vi "Sending U8x2 CMD and String Data.vi"(0 "TCP Ref In":refnum<k5>, 1 "Time Out(ms)":i32=100, 5 "High CMD":u8, 7 "Low CMD":u8, 9 "Data":string, 11 "error in (no error)":errorcluster) -> (4 "TCP Ref Out":refnum<k5>, 15 "error out":errorcluster)   [LabVIEW 2024]
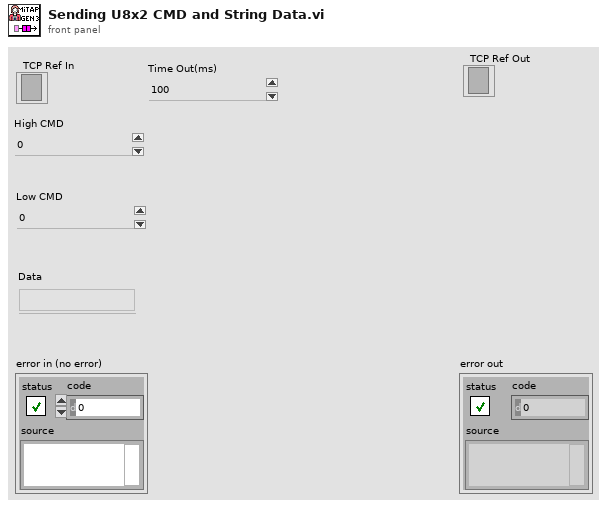
[diagram p1: front panel]
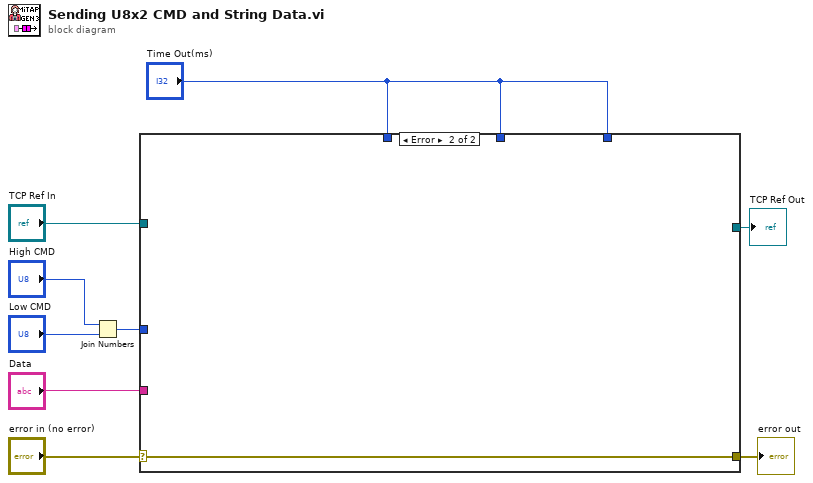
[diagram p0: block diagram]
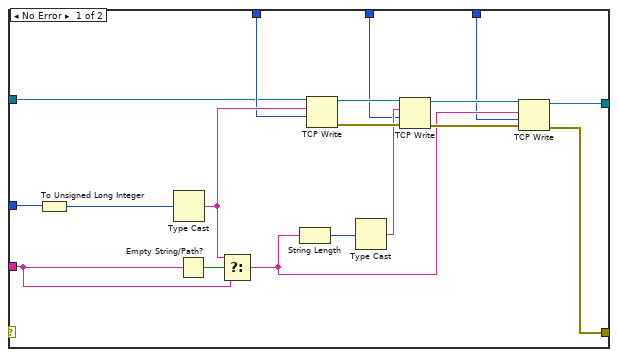
[diagram p2: hidden frame]
diagram:
  n1 = Join Numbers(hi="High CMD", lo="Low CMD") -> ((hi.lo)=w5:u16)
  n2 = case shown="Error" "error in (no error)" {
    selector: "error in (no error)" -> [_ w28]
    tunnel: [w18 w28] -> w9
    tunnel: "Time Out(ms)" -> [w17 _]
    tunnel: "Time Out(ms)" -> [w16 _]
    tunnel: "Time Out(ms)" -> [w15 _]
    tunnel: "TCP Ref In" -> [w14 _]
    tunnel: [w13 _] -> w6
    tunnel: w5 -> [w12 _]
    tunnel: "Data" -> [w10 _]
    frame No Error {
      n3 = To Unsigned Long Integer(number=w12) -> (unsigned 32bit integer=w11:u32)
      n4 = Type Cast(x=w11) -> (*(type *) &x=w20:string)  [unwired: 1 in]
      n5 = Empty String/Path?(string/path=w10) -> (empty?=w21:bool)
      n6 = Select(t=w20, s=w21, f=w10) -> (s? t:f=w19:string)
      n7 = String Length(string=w19) -> (length=w23:i32)
      n8 = TCP Write(connection ID=w14, data in=w20, 9:w17) -> (connection ID out=w27:refnum<k5>, error out=w26:errorcluster)  [unwired: 1 in, 1 out]
      n9 = Type Cast(x=w23) -> (*(type *) &x=w22:string)  [unwired: 1 in]
      n10 = TCP Write(connection ID=w27, data in=w22, error in (no error)=w26, 9:w16) -> (connection ID out=w24:refnum<k5>, error out=w25:errorcluster)  [unwired: 1 out]
      n11 = TCP Write(connection ID=w24, data in=w19, error in (no error)=w25, 9:w15) -> (connection ID out=w13:refnum<k5>, error out=w18:errorcluster)  [unwired: 1 out]
    }
    frame Error {
    }
  }
  "error out" <- w9
  "TCP Ref Out" <- w6
